vi "Send UDP.vi"(6 "Operation":enum16{"Init", "Send", "Close"}(ring)=enum."Send", 7 "remote port":u16=61557, 8 "error in":errorcluster, 10 "Pilot":bool, 11 "local port":u16=61556) -> (0 "error out":errorcluster, 2 "Data out":i32)   [LabVIEW 2021]
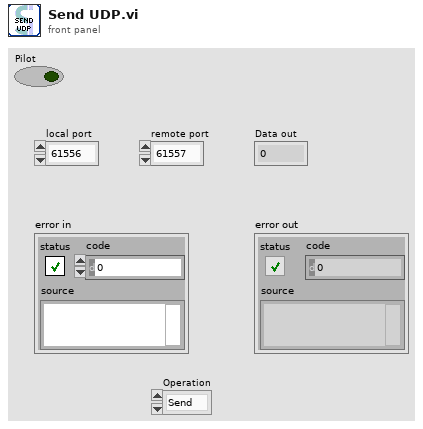
[diagram p1: front panel]
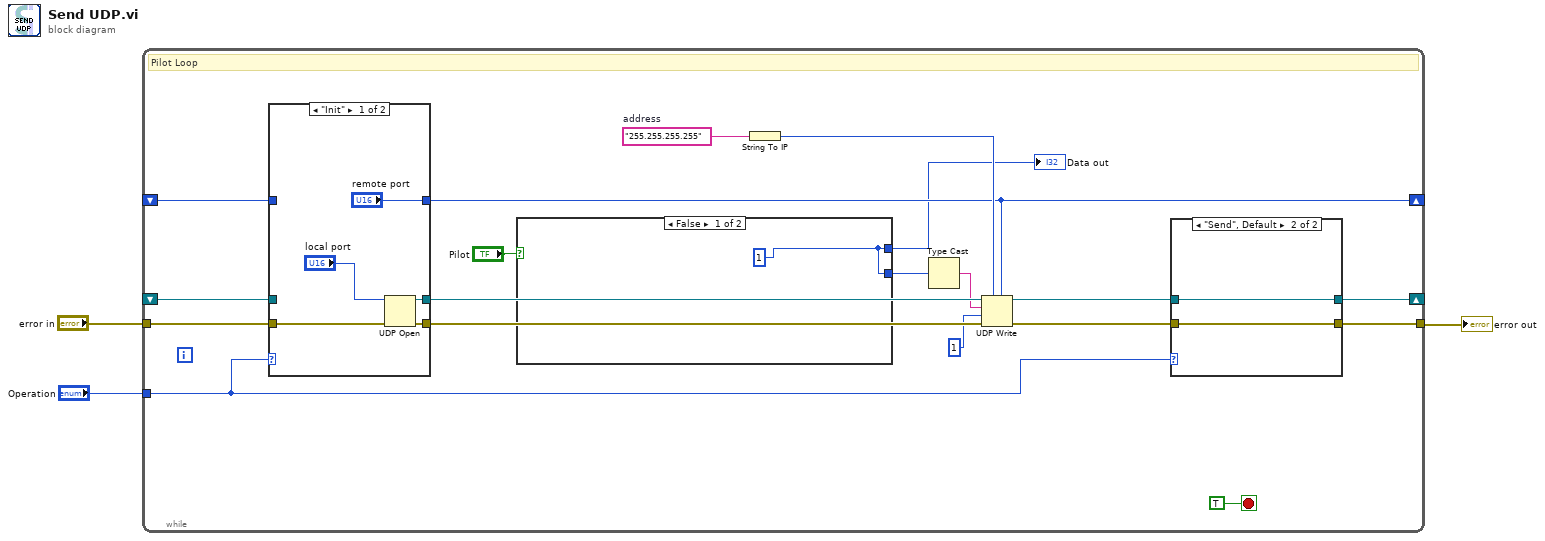
[diagram p0: block diagram]
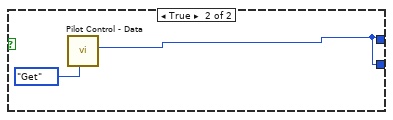
[diagram p2: hidden frame]
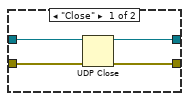
[diagram p3: hidden frame]
diagram:
  n1 = while {
    tunnel: "error in" -> [w21]
    shift-right: [w13] -> _
    shift-left: _ -> [w18]
    tunnel: "Operation" -> [w12]
    tunnel: [w15] -> w1
    shift-right: [w9] -> _
    shift-left: _ -> [w8]
    stop <- TRUE stop-if-true
    w11 = "255.255.255.255"  # address
    # "Pilot Loop"
    n2 = case shown="\"Init\"" w12 {
      tunnel: w21 -> [w33 w38]
      tunnel: [w35 w38] -> w20
      tunnel: [w34 w39] -> w19
      tunnel: w18 -> [_ w39]
      tunnel: ["remote port" w37] -> w9
      tunnel: w8 -> [_ w37]
      frame "Init" {
        n3 = UDP Open(8:w33, 11:"local port") -> (port=w34:refnum<k16>, 0:w35:errorcluster)  [unwired: 3 in, 1 out]
      }
      frame "Send", Default {
      }
    }
    n4 = case shown="False" "Pilot" {
      tunnel: [w23 w24] -> w6
      tunnel: [w23 w24] -> w4
      frame False {
        w23 = 1
      }
      frame True {
        n5 = call "Pilot Control - Data.vi"("Operation"=enum16{"Init", "Get", "Set"}."Get") -> ("Data out"=w24:i32)  [unwired: 10 in]
      }
    }
    "Data out" <- w6
    n6 = String To IP(1:w11) -> (0:w10:u32)
    n7 = Type Cast(x=w4) -> (*(type *) &x=w5:string)  [unwired: 1 out]
    n8 = UDP Write(address=w10, port or service name=w9, connection ID=w19, data in=w5, 8:w20, 9:1 ("timeout ms (25000)")) -> (error out=w16:errorcluster, 3:w14:refnum<k16>)
    n9 = case shown="\"Send\", Default" w12 {
      tunnel: w16 -> [w29 w31]
      tunnel: [w28 w31] -> w15
      tunnel: w14 -> [w27 w30]
      tunnel: [w26 w30] -> w13
      frame "Close" {
        n10 = UDP Close(connection ID=w27, 8:w29) -> (connection ID out=w26:refnum<k16>, error out=w28:errorcluster)
      }
      frame "Send", Default {
      }
    }
  }
  "error out" <- w1
